vi "Fields Delete From Sequence.vi"(8 "error in (no error)":errorcluster, 10 "sxSequenceId (\"\")":string, 11 "Connection Refnum":T1) -> (0 "error out":errorcluster, 3 "Connection Refnum":T1)   [LabVIEW 2011]
uses:
  Summitek EXT/ODBC/SQL Controls/Connection Refnum.ctl
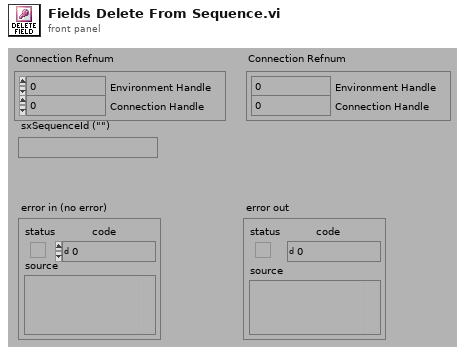
[diagram p1: front panel]
types:
  T1 = typedef "Connection Refnum.ctl" = cluster{"Environment Handle":i32, "Connection Handle":i32}
  T2 = typedef "Statement Refnum.ctl" = cluster{"Statement Handle":i32, "Parameter Number":u16}
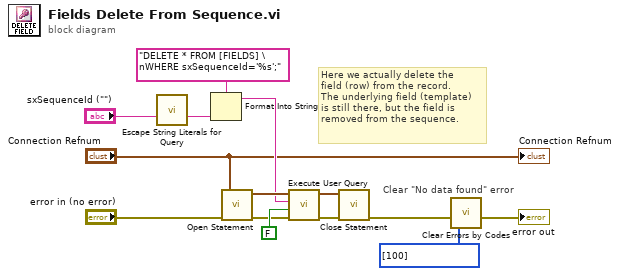
[diagram p0: block diagram]
diagram:
  # "Here we actually delete the\nfield (row) from the record.\nThe underlying field (template)\nis still there, but the field is\nremoved from the sequence."
  # "Clear \"No data found\" error"
  n1 = call "Escape String Literals for Query.vi"("String"="sxSequenceId (\"\")") -> ("escaped String"=w5:string)  [unwired: 1 in, 13 out]
  n2 = Format Into String(format string="DELETE * FROM [FIELDS] \nWHERE sxSequenceId='%s';" ("User Query"), w5) -> (resulting string=w9:string)  [unwired: 2 in, 1 out]
  n3 = call "Open Statement.vi"("error in (no error)"="error in (no error)", "Connection Refnum"="Connection Refnum") -> ("error out"=w11:errorcluster, "Statement Refnum"=w10:T2)  [unwired: 4 out]
  n4 = call "Execute User Query.vi"("error in (no error)"=w11, "Return Data? (f)"=FALSE, "User Query"=w9, "Statement Refnum"=w10) -> ("error out"=w12:errorcluster, "Statement Refnum"=w13:T2)  [unwired: 2 out]
  n5 = call "Close Statement.vi"("error in (no error)"=w12, "Statement Refnum"=w13) -> ("error out"=w8:errorcluster)  [unwired: 5 out]
  n6 = call "Clear Errors by Codes.vi"("Error Codes\nto Clear (Empty)"=i32[] [100] ("Error Codes\nto Clear (Empty)"), "error in (no error)"=w8) -> ("error out"=→"error out":errorcluster)  [unwired: 5 out]
  "Connection Refnum" <- "Connection Refnum"
